vi "NanotecSMCPD.move axis relative.vi"(0 "i ref in":refnum<vi>, 1 "axis":i32, 2 "relPosition":dbl, 3 "ms timeout (10000)":i32=10000, 5 "error in (no error)":errorcluster) -> (14 "i ref out":refnum<vi>, 17 "timed out":bool, 19 "error out":errorcluster)   [LabVIEW 2014, in "NanotecSMCPD.lvlib"]
doc: "Moves the specified axis by the relative position specified."
uses:
  NanotecSMCPD.lvlib
  CS_Core/CSSystem/CoreDefs/CoreDefs.error_type.ctl
  CS_Core/CSSystem/CoreDefs/CoreDefs.error_severity.ctl
  CS_Core/CSApplicationBaseClasses/MotorBase/MotorBase.directionType.ctl
  CS_Core/CSApplicationBaseClasses/MotorBase/MotorBase.serviceType.ctl
  CS_Core/CSApplicationBaseClasses/MotorBase/MotorBase.statusType.ctl
  CSlibraries/UtilityLib/UtilityLib.valueStatus.ctl
  CS_Core/CSApplicationBaseClasses/DeviceBase/DeviceBase.lvlib
  CS_Core/CSSystem/CoreLib/CoreLib.lvlib
  CS_Core/CSApplicationBaseClasses/MotorBase/MotorBase.lvlib
  CSlibraries/UtilityLib/UtilityLib.lvlib
  instr.lib/NanotecSMCPD/NanotecSMCPDDriver.lvlib
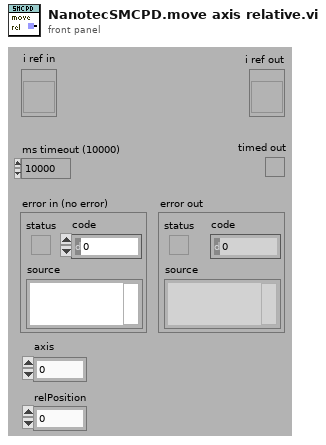
[diagram p1: front panel]
types:
  T1 = typedef "CoreDefs.error_severity.ctl" = enum16{"undefined", "information", "warning", "error", "fatal"}
  T2 = typedef "CoreDefs.error_type.ctl" = enum16{"no error", "can't load process", "can't unload process", "process does not exist", "can't install process", "can't remove process", "unknown function", "time out", "can't execute function", "duplicate queue name", "super not found", "caller queue invalid", "can't ping process", "unknown error", "VISA Error", "VISA timeout", "GPIB timeout", "GPIB error", "communication error", "data type mismatch", "can't read data from OPC server", "can't write data to OPC server", "OET error", "function not implemented", "process already exists", "invalid Shared Variable name", "error writing Shared Variable", "error reading Shared Variable", "invalid client name", "corrupt database", "unknown class", "call not authorized", "parameter out of range", "OET timeout: can't get data to modify", "invalid queue name", "requested operation incompatible with current state", "event undefined", "event disabled", "state undefined", "caller is not a friend", "EventBuilder: bad eventID", "EventBuilder: no DAQ devices", "a thread must not stop itself", "UNUSED ELEMENT4", "DiscArchiver: eventData incomplete", "DiscArchiver: eventData does not belong to run", "DiscArchiver: can't open file", "DiscArchiver: can't write to file", "DiscArchiver: available disc space low", "can't acquire semaphore", "error reading data from database", "notifier object is not existing", "can't register process", "can't unregister process", "illegal event type", "object disabled", "object already exists", "can't change state", "Instrument not found", "no connection to remote node", "invalid reference", "N/A", "UNUSED ELEMENT 1", "element not found", "illegal TCP/IP connection detected", "object does not exist", "invalid access ID", "unknown CS system", "invalid privilige", "unsupported data type", "unsupported server type", "IO server already exists", "Shared Variable already exists"}
  T3 = typedef "UtilityLib.lvlib/UtilityLib.valueStatus.ctl" = enum16{"no info available", "stand by/off", "on", "warning", "alarm/malfunction", "not implemented", "user action required", "important information", "system default", "control default", "indicator default", "button default"}
  T4 = typedef "MotorBase.lvlib/MotorBase.serviceType.ctl" = enum16{"onOff", "startVelocity", "stopVelocity", "acceleration", "rangeMin", "rangeMax", "status", "position"}
  T5 = typedef "MotorBase.lvlib/MotorBase.directionType.ctl" = enum16{"unknown", "update actual value", "update nominal value", "update both"}
  T6 = typedef "MotorBase.lvlib/MotorBase.statusType.ctl" = u32
  T7 = typedef "NanotecSMCPD.lvlib/NanotecSMCPD.i attribute.ctl" = cluster{"referencing":bool[], "stop":bool[], "AutoHalt ID":i32, "MethodQueue":refnum<queue>, "Referenced1Time?":bool[], "LastCommand ID":i32}
  T8 = typedef "MotorBase.lvlib/MotorBase.i attribute.ctl" = cluster{"defaultAxisIndex":i32, "logicalName":string[], "nOfAxes":i32, "physicalName":string[], "scaling":dbl[], "units":string[], "defaulAxisIndexID":i32, "logicalNameID":i32, "nOfAxesID":i32, "physicalNameID":i32, "unitID":i32, "actValues":T9, "nomValues":T9}
  T9 = typedef "MotorBase.lvlib/MotorBase.parameters.ctl" = cluster{"services":cluster{"onOff":bool[], "startVelocity":dbl[], "stopVelocity":dbl[], "acceleration":dbl[], "rangeMin":dbl[], "rangeMax":dbl[], "status":T6[], "position":dbl[]}, "serviceIDs":cluster{"onOffID":i32, "startVelocityID":i32, "stopVelocityID":i32, "accelerationID":i32, "rangeMinID":i32, "rangeMaxID":i32, "statusID":i32, "positionID":i32}}
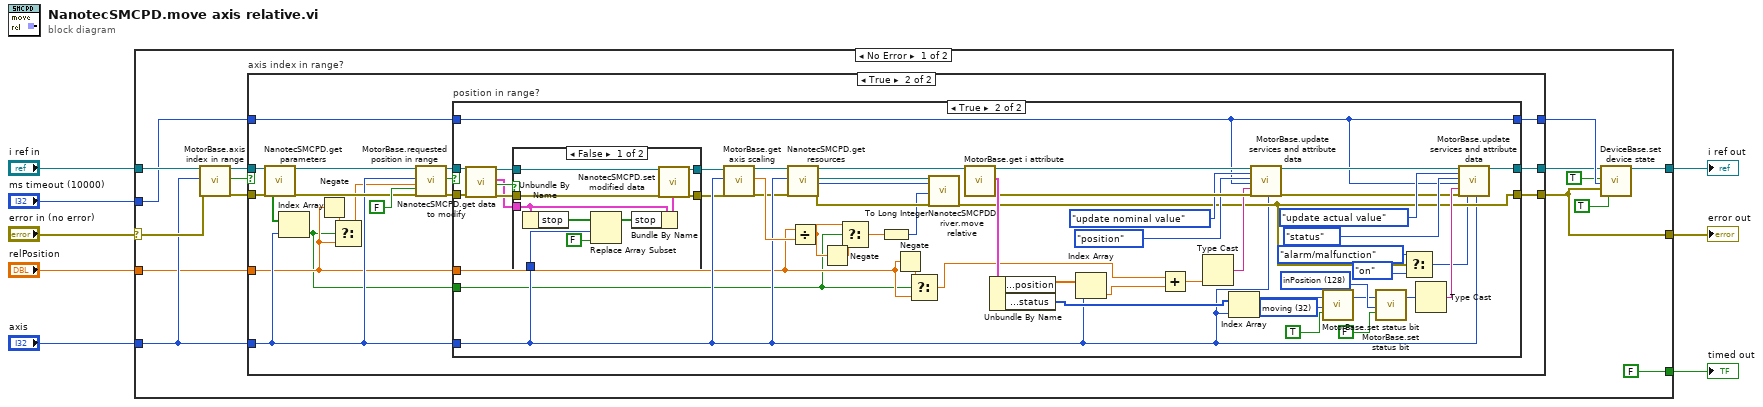
[diagram p0: block diagram]
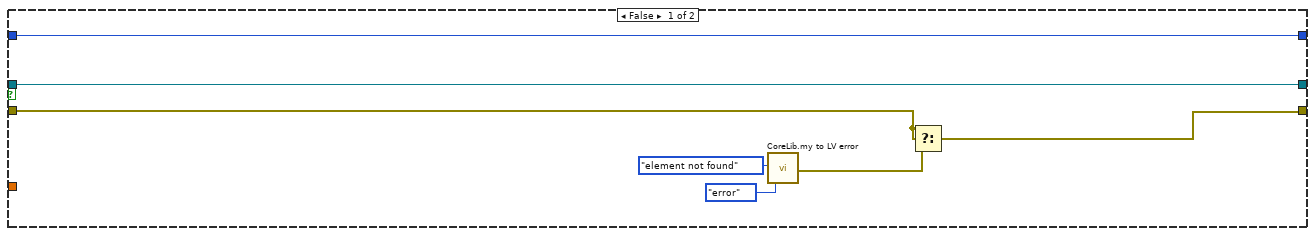
[diagram p2: hidden frame]
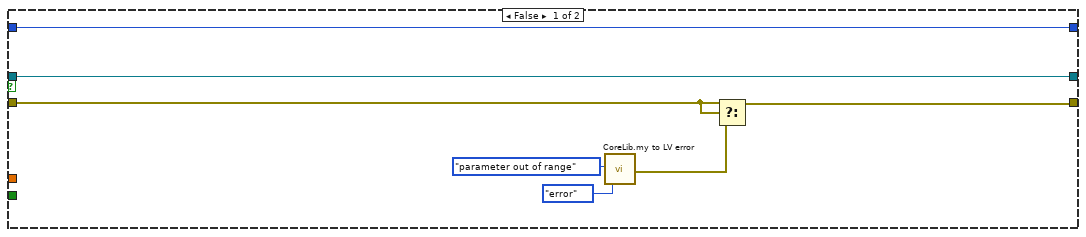
[diagram p3: hidden frame]
diagram:
  n1 = case shown="No Error" "error in (no error)" {
    selector: "error in (no error)" -> [w16 w120]
    tunnel: "ms timeout (10000)" -> [w13 _]
    tunnel: "i ref in" -> [w17 w121]
    tunnel: [w15 w120] -> w5
    tunnel: "axis" -> [w14 _]
    tunnel: [w12 w121] -> w3
    tunnel: "relPosition" -> [w11 _]
    tunnel: [FALSE _] -> w1
    frame No Error {
      n2 = call "MotorBase.axis index in range.vi"("i ref in"=w17, "axisIndex"=w14, "error in (no error)"=w16) -> ("i ref out"=w21:refnum<vi>, "in range"=w20:bool, "error out"=w22:errorcluster)  [unwired: 14 in]
      n3 = case "axis index in range?" shown="True" w20 {
        tunnel: [w30 w48] -> w19
        tunnel: [w27 w47] -> w15
        tunnel: w13 -> [w24 w46]
        tunnel: w14 -> [_ w35]
        tunnel: w21 -> [w30 w40]
        tunnel: w22 -> [w28 w39]
        tunnel: [w24 w42] -> w23
        tunnel: w11 -> [_ w34]
        frame False {
          n4 = call "CoreLib.my to LV error.vi"("ErrorTypes"=CoreDefs.error_type."element not found", "severityLevel"=CoreDefs.error_severity."error") -> ("myErrorCluster"=w26:errorcluster)  [unwired: 16 in, 1 out]
          n5 = Select(t=w28, s=w28, f=w26) -> (s? t:f=w27:errorcluster)
        }
        frame True {
          n6 = call "NanotecSMCPD.get parameters.vi"("i ref in"=w40, "error in (no error)"=w39) -> ("ReverseDirection?"=w36:bool[], "i ref out"=w38:refnum<vi>, "error out"=w37:errorcluster)  [unwired: 6 in, 9 out]
          n7 = Index Array(array=w36, index=w35) -> (element=w31:bool)
          n8 = Negate(x=w34) -> (-x=w33:dbl)
          n9 = Select(t=w33, s=w31, f=w34) -> (s? t:f=w32:dbl)
          n10 = call "MotorBase.requested position in range.vi"("i ref in"=w38, "axisIndex"=w35, "reqPosition"=w32, "absolute"=FALSE, "error in (no error)"=w37) -> ("i ref out"=w44:refnum<vi>, "in range"=w45:bool, "error out"=w43:errorcluster)  [unwired: 12 in]
          n11 = case "position in range?" shown="True" w45 {
            tunnel: w44 -> [w52 w67]
            tunnel: w43 -> [w51 w68]
            tunnel: [w52 w106] -> w48
            tunnel: [w50 w84] -> w47
            tunnel: w46 -> [w49 w74]
            tunnel: w35 -> [_ w69]
            tunnel: w34 -> [_ w61]
            tunnel: [w49 w74] -> w42
            tunnel: w31 -> [_ w56]
            frame False {
              n12 = call "CoreLib.my to LV error.vi"("ErrorTypes"=CoreDefs.error_type."parameter out of range", "severityLevel"=CoreDefs.error_severity."error") -> ("myErrorCluster"=w54:errorcluster)  [unwired: 16 in, 1 out]
              n13 = Select(t=w51, s=w51, f=w54) -> (s? t:f=w50:errorcluster)
            }
            frame True {
              w76 = T6 32 items=["motorEnabled"=1, "negativeLimitSwitchActive"=2, "positiveLimitSwitchActive"=4, "limitSwitchesEnabled"=8, "limitSwitchesAreNormallyClosed"=16, "moving"=32, "referenced"=64, "inPosition"=128, "reserved2"=256, "reserved3"=512, "reserved4"=1024, "reserved5"=2048, "error"=4096, "reserved6"=8192, "reserved7"=16384, "reserved8"=32768, "user defined1"=65536, "user defined2"=131072, "user defined3"=262144, "user defined4"=524288, "user defined5"=1048576, "user defined6"=2097152, "user defined7"=4194304, "user defined8"=8388608, "user defined9"=16777216, "user defined10"=33554432, "user defined11"=67108864, "user defined12"=134217728, "user defined13"=268435456, "user defined14"=536870912, "user defined15"=1073741824, "user defined16"=2147483648] ("statusBit")
              w87 = T6 128 items=["motorEnabled"=1, "negativeLimitSwitchActive"=2, "positiveLimitSwitchActive"=4, "limitSwitchesEnabled"=8, "limitSwitchesAreNormallyClosed"=16, "reseved1"=32, "referenced"=64, "inPosition"=128, "reserved2"=256, "reserved3"=512, "reserved4"=1024, "reserved5"=2048, "error"=4096, "reserved6"=8192, "reserved7"=16384, "reserved8"=32768, "user defined1"=65536, "user defined2"=131072, "user defined3"=262144, "user defined4"=524288, "user defined5"=1048576, "user defined6"=2097152, "user defined7"=4194304, "user defined8"=8388608, "user defined9"=16777216, "user defined10"=33554432, "user defined11"=67108864, "user defined12"=134217728, "user defined13"=268435456, "user defined14"=536870912, "user defined15"=1073741824, "user defined16"=2147483648] ("service")
              n14 = call "NanotecSMCPD.get data to modify.vi"("i ref in"=w67, "error in (no error)"=w68) -> ("i ref out"=w72:refnum<vi>, "i attribute"=w70:T7, "timed out"=w73:bool, "error out"=w71:errorcluster)  [unwired: 14 in]
              n15 = case shown="False" w73 {
                tunnel: w72 -> [w117 w119]
                tunnel: [w116 w119] -> w66
                tunnel: w71 -> [w115 w118]
                tunnel: [w114 w118] -> w65
                tunnel: w70 -> [w113 _]
                tunnel: w69 -> [w109 _]
                frame False {
                  n16 = Unbundle By Name(w113) -> ("stop"=w111:bool[])
                  n17 = Replace Array Subset(array=w111, new element=FALSE ("new element/subarray"), index=w109) -> (w110:bool[])
                  n18 = Bundle By Name(cluster=w113, "stop"=w110) -> (w112:T7)
                  n19 = call "NanotecSMCPD.set modified data.vi"("i ref in"=w117, "i attribute"=w112, "error in (no error)"=w115) -> ("i ref out"=w116:refnum<vi>, "error out"=w114:errorcluster)  [unwired: 15 in]
                }
                frame True {
                }
              }
              n20 = call "MotorBase.get axis scaling.vi"("i ref in"=w66, "axisIndex"=w69, "error in (no error)"=w65) -> ("i ref out"=w64:refnum<vi>, "scaling"=w85:dbl, "error out"=w63:errorcluster)  [unwired: 14 in]
              n21 = call "NanotecSMCPD.get resources.vi"("i ref in"=w64, "axisNumber"=w69, "error in (no error)"=w63) -> ("i ref out"=w89:refnum<vi>, "VISA resource"=w91:refnum<visa-resource-name>, "address"=w80:i32, "error out"=w90:errorcluster)  [unwired: 13 in]
              n22 = Divide(x=w61, y=w85) -> (x/y=w57:dbl)
              n23 = Negate(x=w57) -> (-x=w58:dbl)
              n24 = Select(t=w57, s=w56, f=w58) -> (s? t:f=w59:dbl)
              n25 = To Long Integer(number=w59) -> (32bit integer=w79:i32)
              n26 = Negate(x=w61) -> (-x=w62:dbl)
              n27 = Select(t=w62, s=w56, f=w61) -> (s? t:f=w60:dbl)
              n28 = call "NanotecSMCPDDriver.move relative.vi"("VISA resource name"=w91, "contollerID"=w80, "nOfSteps [uSteps]"=w79, "error in (no error)"=w90) -> ("error out"=w84:errorcluster)  [unwired: 13 in, 2 out]
              n29 = call "MotorBase.get i attribute.vi"("i ref in"=w89) -> ("i ref out"=w102:refnum<vi>, "i attribute"=w103:T8, "error out"=w99:errorcluster)  [unwired: 16 in]
              n30 = Unbundle By Name(w103) -> ("actValues.services.position"=w94:dbl[], "actValues.services.status"=w95:T6[])
              n31 = Index Array(array=w94, index=w69) -> (element=w93:dbl)
              n32 = Add(x=w60, y=w93) -> (x+y=w92:dbl)
              n33 = Type Cast(x=w92) -> (*(type *) &x=w98:string)  [unwired: 1 in]
              n34 = Index Array(array=w95, index=w69) -> (element=w78:T6)
              n35 = call "MotorBase.update services and attribute data.vi"("i ref in"=w102, "direction"=MotorBase.directionType."update nominal value", "service"=MotorBase.serviceType."position", "ms timeout (10000)"=w74, "value"=w98, "error in (no error)"=w99, "axisNumber"=w69) -> ("i ref out"=w101:refnum<vi>, "error out"=w100:errorcluster)  [unwired: 10 in, 1 out]
              n36 = call "MotorBase.set status bit.vi"("status"=w78, "statusBit"=w76, "setBit"=TRUE) -> ("status out"=w77:T6)  [unwired: 16 in]
              n37 = call "MotorBase.set status bit.vi"("status"=w77, "statusBit"=w87, "setBit"=FALSE) -> ("status out"=w88:T6)  [unwired: 16 in]
              n38 = Select(t=UtilityLib.valueStatus."alarm/malfunction", s=w84, f=UtilityLib.valueStatus."on" ("quality")) -> (s? t:f=w81:T3)
              n39 = Type Cast(x=w88) -> (*(type *) &x=w107:string)  [unwired: 1 in]
              n40 = call "MotorBase.update services and attribute data.vi"("i ref in"=w101, "direction"=MotorBase.directionType."update actual value", "service"=MotorBase.serviceType."status", "ms timeout (10000)"=w74, "value"=w107, "error in (no error)"=w100, "quality"=w81, "axisNumber"=w69) -> ("i ref out"=w106:refnum<vi>)  [unwired: 9 in, 2 out]
            }
          }
        }
      }
      n41 = call "DeviceBase.set device state.vi"("i ref in"=w19, "implicit"=TRUE, "ms timeout (10000)"=w23, "device error"=w15, "mayResetError (FALSE)"=TRUE) -> ("i ref out"=w12:refnum<vi>)  [unwired: 12 in, 2 out]
    }
    frame Error {
    }
  }
  "error out" <- w5
  "i ref out" <- w3
  "timed out" <- w1
